vi "ComapreLaserVariablesScannerRead.vi"(9 "ScanerReadOut":string[](array[string]), 11 "LaserVariables":string[](array[string])) -> (2 "Equals?":bool, 3 "String":string)   [LabVIEW 2016]
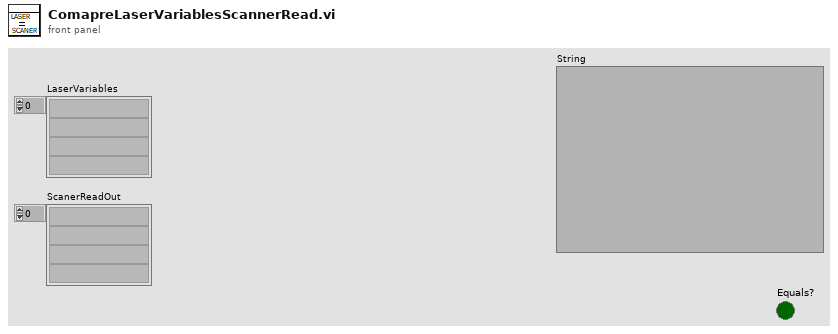
[diagram p1: front panel]
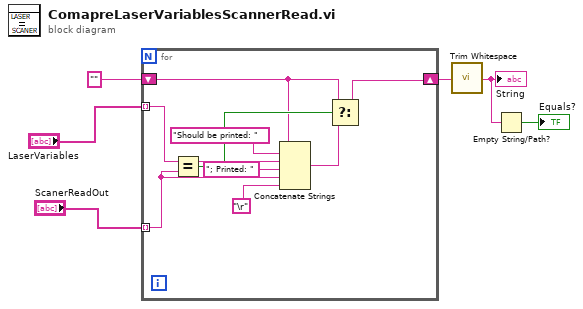
[diagram p0: block diagram]
diagram:
  n1 = for {
    tunnel: "LaserVariables" -> [w12] mode=indexing
    tunnel: "ScanerReadOut" -> [w10] mode=indexing
    shift-right: [w14] -> w3
    shift-left: "" -> [w7]
    n2 = Equal?(x=w12, y=w10) -> (x = y?=w15:bool)
    n3 = Concatenate Strings(w7, "Should be printed: " ("string"), w12, "; Printed: " ("string"), w10, "\r") -> (w9:string)
    n4 = Select(t=w7, s=w15, f=w9) -> (s? t:f=w14:string)
  }
  n5 = call <vilib>:"Trim Whitespace.vi"("string"=w3) -> ("trimmed string"=w2:string)  [unwired: 1 in]
  "String" <- w2
  n6 = Empty String/Path?(string/path=w2) -> (empty?=→"Equals?":bool)
